vi "Open Config File and check version.vi"(7 "Version String":string, 8 "error in":errorcluster, 11 "Ini path":path) -> (0 "error out":errorcluster, 1 "file created?":bool, 2 "Version changed?":bool, 3 "refnum":T1)   [LabVIEW 2009, in "FileIO lib.lvlib"]
doc: "Opens or creates an in i file at the specified path. Shecks the version string [Application] Version = 'string'.\nReturns an error if file can not be creates, returns a warning if file is new or version string has changed."
uses:
  <vilib>/Utility/config.llb/Config Data RefNum.ctl
  FileIO lib.lvlib
  <vilib>/Utility/config.llb/NI_LVConfig.lvlib
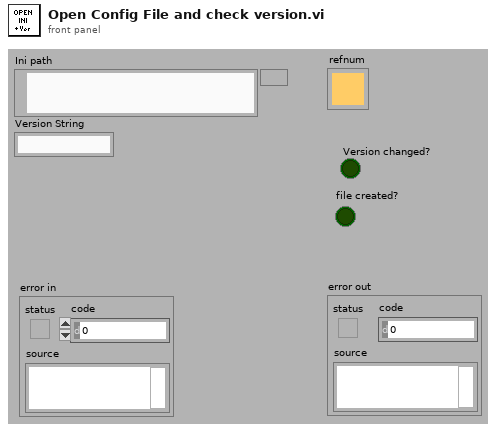
[diagram p1: front panel]
types:
  T1 = typedef "NI_LVConfig.lvlib/Config Data RefNum.ctl" = refnum<k1>
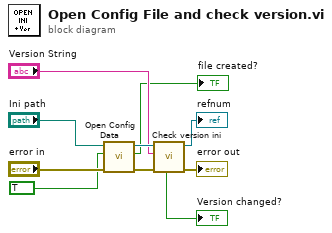
[diagram p0: block diagram]
diagram:
  n1 = call <vilib>:"Open Config Data.vi"("error in (no error)"="error in", "create file if necessary (T)"=TRUE, "configuration file path"="Ini path") -> ("error out"=w8:errorcluster, "file created?"=→"file created?":bool, "refnum"=w7:T1)  [unwired: 6 in]
  n2 = call "Check version ini.vi"("error in"=w8, "Version String"="Version String", "refnum in"=w7) -> ("error out"=→"error out":errorcluster, "refnum"=→"refnum":T1, "Version changed"=→"Version changed?":bool)  [unwired: 6 in]
